vi "前面板对象数据接收.vi"() -> ()   [LabVIEW 2010]
panel:
  in  "幅度控制":dbl(knob) scale=0.0..10.0
  in  "stop":bool
  out "波形接收":dbl[](graph)
  # "1.按照教材要求修改各个控件链接的URL\n2.打开DataSocket Server\n3.运行前面板对象数据传递VI\n4.运行此VI\n5.幅度控制钮可以调整两个VI的正弦波幅值\n6.停止控制钮可以使两个VI停下来"
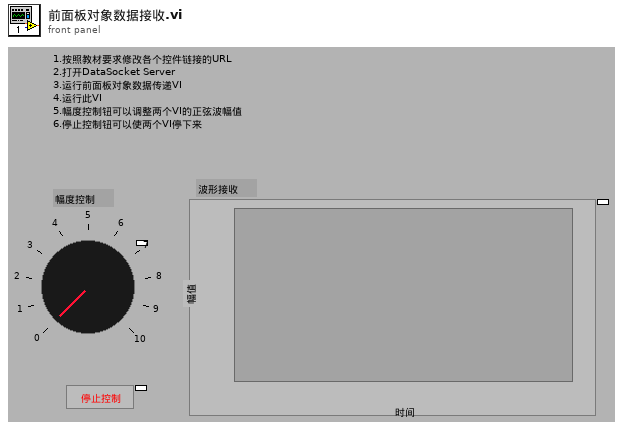
[diagram p1: front panel]
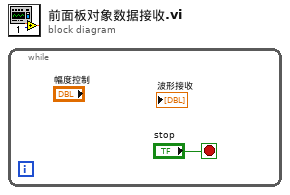
[diagram p0: block diagram]
diagram:
  n1 = while {
    stop <- "stop" stop-if-true
  }
